vi "DestroyCommunication.vi"(8 "error in (no error)":errorcluster, 11 "Message Queues out":T1) -> (0 "error out":errorcluster)   [LabVIEW 2017, in "Server.lvlib" / "Message Queue.lvlib"]
doc: "Destroys all Queues and User Events."
uses:
  Message Queue.lvlib
  CommReferences.ctl
  MessageCluster.ctl
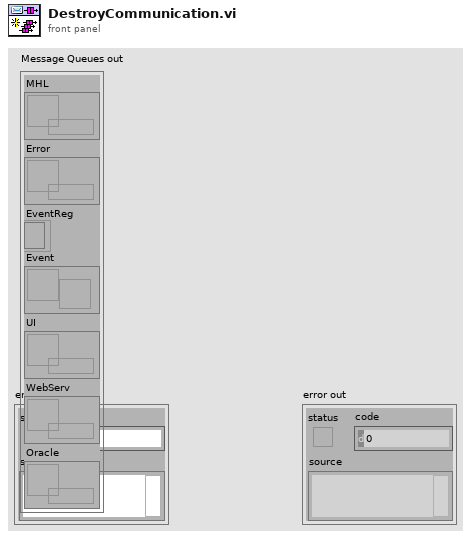
[diagram p1: front panel]
types:
  T1 = typedef "Server.lvlib/Message Queue.lvlib/CommReferences.ctl" = cluster{"MHL":refnum<queue>, "Error":refnum<queue>, "EventReg":refnum<event-registration>, "Event":refnum<user-event>, "UI":refnum<queue>, "WebServ":refnum<queue>, "Oracle":refnum<queue>}
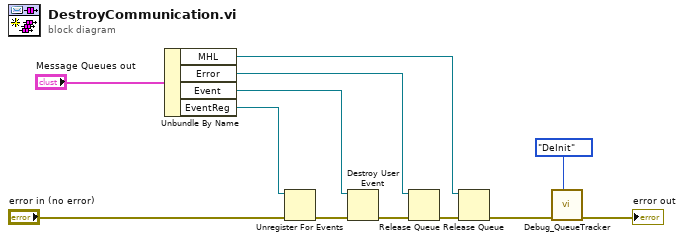
[diagram p0: block diagram]
diagram:
  n1 = Unbundle By Name("Message Queues out") -> ("MHL"=w3:refnum<queue>, "Error"=w5:refnum<queue>, "Event"=w7:refnum<user-event>, "EventReg"=w9:refnum<event-registration>)
  n2 = Unregister For Events(event registration refnum=w9, error in="error in (no error)") -> (error out=w10:errorcluster)
  n3 = Destroy User Event(user event=w7, error in=w10) -> (error out=w8:errorcluster)
  n4 = Release Queue(queue=w5, error in (no error)=w8) -> (error out=w6:errorcluster)  [unwired: 1 in, 2 out]
  n5 = Release Queue(queue=w3, error in (no error)=w6) -> (error out=w4:errorcluster)  [unwired: 1 in, 2 out]
  n6 = call "Debug_QueueTracker.vi"("Mode"=enum16{"Init", "Track", "DeInit"}."DeInit", "Error In"=w4) -> ("Error Out"=→"error out":errorcluster)  [unwired: 9 in]
